vi "Read This VI.vi"(8 "error in (no error)":errorcluster, 11 "Coca Actor in":refnum<class "Coca Actor.lvclass">) -> (0 "error out":errorcluster, 2 "This VI":refnum<vi>, 3 "Coca Actor out":refnum<class "Coca Actor.lvclass">)   [LabVIEW 2020, in "Coca Actor.lvlib" / "Coca Actor.lvclass"]
uses:
  Coca Actor.lvclass
  Coca Actor.lvclass/Coca Actor.ctl
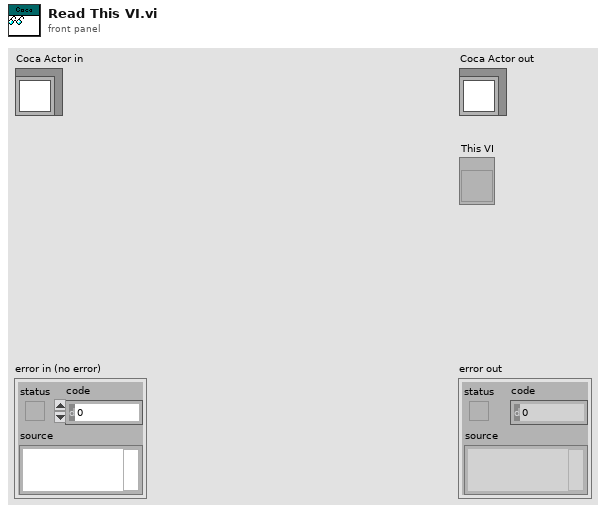
[diagram p1: front panel]
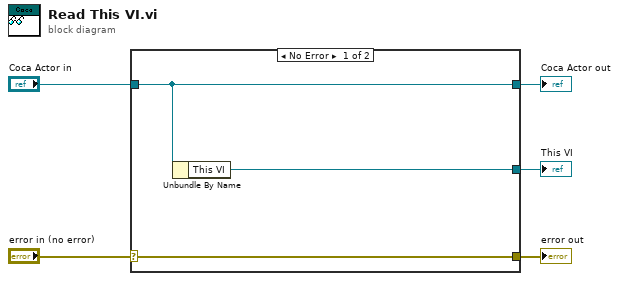
[diagram p0: block diagram]
diagram:
  n1 = case shown="No Error" "error in (no error)" {
    selector: "error in (no error)" -> [w8 w9]
    tunnel: [w8 w9] -> w4
    tunnel: [w7 w10] -> w2
    tunnel: "Coca Actor in" -> [w7 w10]
    tunnel: [w6 _] -> w1
    frame No Error {
      n2 = Unbundle By Name(w7) -> ("This VI"=w6:refnum<vi>)
    }
    frame Error {
    }
  }
  "error out" <- w4
  "Coca Actor out" <- w2
  "This VI" <- w1
